vi "Read Content.vi"(8 "Error In":errorcluster, 11 "Tag In":refnum<class "Tag.lvclass">) -> (0 "Error Out":errorcluster, 2 "Content":string, 3 "Tag Out":refnum<class "Tag.lvclass">)   [LabVIEW 2018, in "Toolkit.lvlib" / "Nodes.lvlib" / "Tag.lvclass"]
uses:
  Tag.lvclass
  NonTerminal/NonTerminal.lvclass
  Tag.lvclass/Tag.ctl
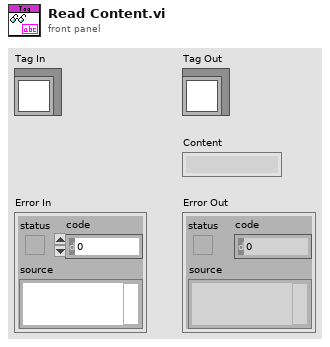
[diagram p1: front panel]
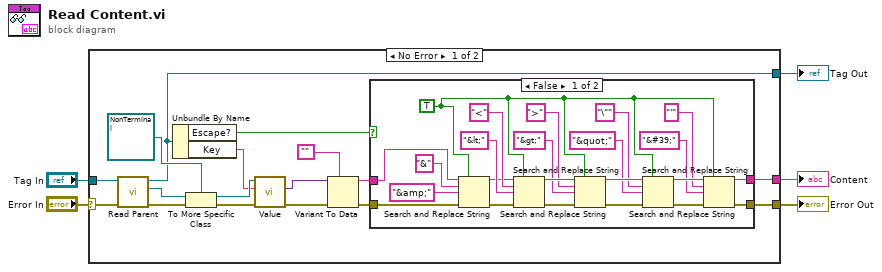
[diagram p0: block diagram]
diagram:
  n1 = case shown="No Error" "Error In" {
    selector: "Error In" -> [w21 w48]
    tunnel: "Tag In" -> [w22 w49]
    tunnel: [w15 w49] -> w3
    tunnel: [w8 w48] -> w2
    tunnel: [w7 _] -> w1
    frame No Error {
      n2 = call-dynamic "Read Parent.vi"("Error In"=w21, "Terminal In"=w22) -> ("Error Out"=w20:errorcluster, "Parent"=w19:refnum<class "Abstract.lvclass">, "Terminal Out"=w15:refnum<class "Tag.lvclass">)  [unwired: 7 in]
      n3 = Unbundle By Name(w15) -> ("Escape?"=w6:bool, "Key"=w14:string)
      n4 = To More Specific Class(target class=refnum<class "NonTerminal.lvclass"> refnum ("Toolkit.lvlib:Nodes.lvlib:NonTerminal.lvclass"), reference=w19, error in=w20) -> (specific class reference=w17:refnum<class "NonTerminal.lvclass">, error out=w16:errorcluster)
      n5 = call-dynamic "Value.vi"("Error In"=w16, "Key"=w14, "Non-Terminal In"=w17) -> ("Error Out"=w13:errorcluster, "Value"=w12:variant)  [unwired: 6 in, 1 out]
      n6 = Variant To Data(error in=w13, type="", Variant=w12) -> (data=w10:string, error out=w9:errorcluster)
      n7 = case shown="False" w6 {
        tunnel: w10 -> [w43 w47]
        tunnel: w9 -> [w42 w46]
        tunnel: [w24 w46] -> w8
        tunnel: [w23 w47] -> w7
        frame False {
          w27 = TRUE ("replace all? (F)")
          n8 = Search and Replace String(replace all?=w27, input string=w43, search string="&", replace string="&amp;" ("replace string (\"\")"), error in=w42) -> (result string=w39:string, error out=w38:errorcluster)  [unwired: 3 in, 2 out]
          n9 = Search and Replace String(replace all?=w27, input string=w39, search string="<", replace string="&lt;" ("replace string (\"\")"), error in=w38) -> (result string=w36:string, error out=w37:errorcluster)  [unwired: 3 in, 2 out]
          n10 = Search and Replace String(replace all?=w27, input string=w36, search string=">", replace string="&gt;" ("replace string (\"\")"), error in=w37) -> (result string=w32:string, error out=w33:errorcluster)  [unwired: 3 in, 2 out]
          n11 = Search and Replace String(replace all?=w27, input string=w32, search string="\"" ("replace string (\"\")"), replace string="&quot;" ("replace string (\"\")"), error in=w33) -> (result string=w29:string, error out=w28:errorcluster)  [unwired: 3 in, 2 out]
          n12 = Search and Replace String(replace all?=w27, input string=w29, search string="'", replace string="&#39;" ("replace string (\"\")"), error in=w28) -> (result string=w23:string, error out=w24:errorcluster)  [unwired: 3 in, 2 out]
        }
        frame True {
        }
      }
    }
    frame Error {
    }
  }
  "Error Out" <- w2
  "Tag Out" <- w3
  "Content" <- w1
